vi "Text as Encoded String (LabVIEW Path).vi"(9 "error in":errorcluster, 10 "Text":path) -> (1 "error out":errorcluster, 2 "Encoded String":T1)   [LabVIEW 2020, in "G-Unicode.lvlib"]
doc: "Converts the input string or path to a raw UTF-8 encoded LabVIEW string. Valid inputs are a UTF-8 String class, UTF-8 Path class, LabVIEW string, or LabVIEW path."
uses:
  G-Unicode.lvlib
  Types/Encoded UTF-8 String.ctl
  Text to UTF-8 (LabVIEW String).vi
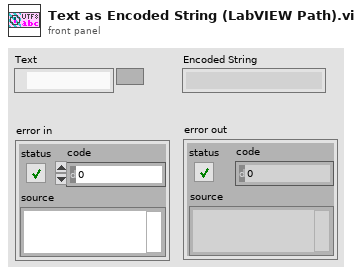
[diagram p1: front panel]
types:
  T1 = typedef "G-Unicode.lvlib/Encoded UTF-8 String.ctl" = string
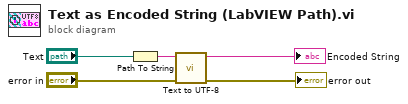
[diagram p0: block diagram]
diagram:
  n1 = Path To String(path="Text") -> (string=w1:string)
  n2 = call-poly "Text to UTF-8.vi"("error in"="error in", "String"=w1) -> ("error out"=→"error out":errorcluster, "UTF-8 Encoded String"=→"Encoded String":T1)  [unwired: 8 in]
